vi "_AboutDialog.vi"(10 "libsAndLicenseInfo in":string, 11 "applicationInfo in":string) -> ()   [LabVIEW 2010]
doc: "A generic 'about' dialog.\nATTENTION: A VI becomes the 'about' dialog if its name starts with 'About'. An underscore '_' as first character avoids that.\n\nCopyright (c) 2018, Martin Weiss\nAll rights reserved.\n\nRedistribution and use in source and binary forms, with or without modification, are permitted provided that the following conditions are met:\n\n1. Redistributions of source code must retain the above copyright notice, this list of conditions and the following disclaimer.\n\n2. Redistributions in binary form must reproduce the above copyright notice, this list of conditions and the following disclaimer in the documentation and/or other materials provided with the distribution.\n\nTHIS SOFTWARE IS PROVIDED BY THE COPYRIGHT HOLDERS AND CONTRIBUTORS \"AS IS\" AND ANY EXPRESS OR IMPLIED WARRANTIES, INCLUDING, BUT NOT LIMITED TO, THE IMPLIED WARRANTIES OF MERCHANTABILITY AND FITNESS FOR A PARTICULAR PURPOSE ARE DISCLAIMED. IN NO EVENT SHALL THE COPYRIGHT HOLDER OR CONTRIBUTORS BE LIABLE FOR ANY DIRECT, INDIRECT, INCIDENTAL, SPECIAL, EXEMPLARY, OR CONSEQUENTIAL DAMAGES (INCLUDING, BUT NOT LIMITED TO, PROCUREMENT OF SUBSTITUTE GOODS OR SERVICES; LOSS OF USE, DATA, OR PROFITS; OR BUSINESS INTERRUPTION) HOWEVER CAUSED AND ON ANY THEORY OF LIABILITY, WHETHER IN CONTRACT, STRICT LIABILITY, OR TORT (INCLUDING NEGLIGENCE OR OTHERWISE) ARISING IN ANY WAY OUT OF THE USE OF THIS SOFTWARE, EVEN IF ADVISED OF THE POSSIBILITY OF SUCH DAMAGE."
uses:
  StyledText/StyledText.lvlib
panel:
  in  "Tab":enum32{"Application", "Libraries"}(tab)
  out "LibsAndLicenses":string caption="Libraries and licenses used by this application"
  in  "OK Button":bool
  # "About"
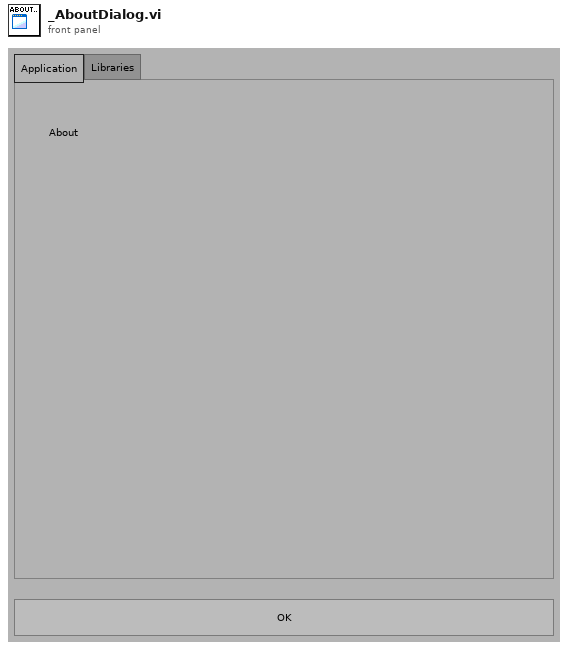
[diagram p1: front panel]
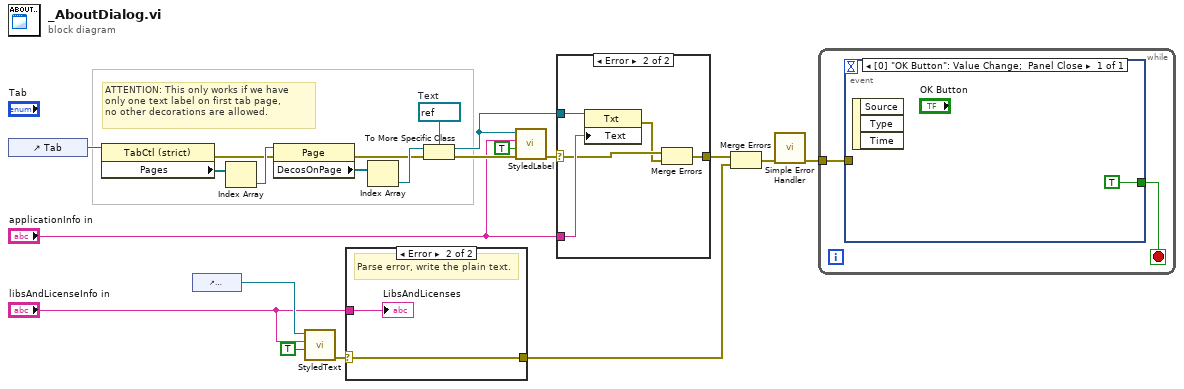
[diagram p0: block diagram]
diagram:
  w19 = refnum<vi> refnum  # Text
  # "ATTENTION: This only works if we have\nonly one text label on first tab page,\nno other decorations are allowed."
  n1 = control-ref of="Tab"() -> (w21:refnum<vi>)
  n2 = property class="TabCtl (strict)"(reference=w21) -> (error out=w14:errorcluster, "Pages"=w20:refnum<vi>[])  [unwired: 1 in, 1 out]
  n3 = control-ref of="LibsAndLicenses"() -> (w17:refnum<vi>)
  n4 = Index Array(array=w20) -> (element=w15:refnum<vi>)  [unwired: 1 in]
  n5 = property class="Page"(reference=w15, error in=w14) -> (error out=w11:errorcluster, "DecosOnPage"=w13:refnum<vi>[])  [unwired: 1 out]
  n6 = call "StyledText.vi"("deferPanelUpdates in"=TRUE, "text in"="libsAndLicenseInfo in", "StringControl"=w17) -> ("error out"=w10:errorcluster)  [unwired: 8 in]
  n7 = case shown="Error" w10 {
    selector: w10 -> [w22 w23]
    tunnel: "libsAndLicenseInfo in" -> [_ w24]
    tunnel: [w22 w23] -> w8
    frame No Error {
    }
    frame Error {
      # "Parse error, write the plain text."
      "LibsAndLicenses" <- w24
    }
  }
  n8 = Index Array(array=w13) -> (element=w12:refnum<vi>)  [unwired: 1 in]
  n9 = To More Specific Class(target class=w19, reference=w12, error in=w11) -> (specific class reference=w6:refnum<vi>, error out=w18:errorcluster)
  n10 = call "StyledLabel.vi"("error in (no error)"=w18, "deferPanelUpdates in"=TRUE, "text in"="applicationInfo in", "Label"=w6) -> ("error out"=w7:errorcluster)  [unwired: 7 in]
  n11 = case shown="Error" w7 {
    selector: w7 -> [w25 w28]
    tunnel: w6 -> [_ w30]
    tunnel: "applicationInfo in" -> [_ w29]
    tunnel: [w25 w26] -> w4
    frame No Error {
    }
    frame Error {
      n12 = property class="Txt"(reference=w30, "Text"=w29) -> (error out=w27:errorcluster)  [unwired: 1 in, 1 out]
      n13 = Merge Errors(w28, w27) -> (w26:errorcluster)
    }
  }
  n14 = Merge Errors(w4, w8) -> (w3:errorcluster)
  n15 = call <vilib>:"Simple Error Handler.vi"("error in (no error)"=w3) -> ("error out"=w16:errorcluster)  [unwired: 4 in, 4 out]
  n16 = while {
    tunnel: w16 -> [w32]
    stop <- w31 stop-if-true
    n17 = event shown="[0] \"OK Button\": Value Change;  Panel Close" {
      selector: _ -> [_]
      dyn-events: _ -> [_]
      timeout: _ -> [_]
      tunnel: w32 -> [_]
      tunnel: [TRUE] -> w31
      event "OK Button": Value Change; Panel Close {
        n18 = event-data() -> ()  [unwired: 1 in, 3 out]
      }
    }
  }
